vi "Read TReading.vi"(8 "error in (no error)":errorcluster, 11 "CameraSession in":refnum<class "CameraSession.lvclass">) -> (0 "error out":errorcluster, 2 "TReading":i16, 3 "CameraSession out":refnum<class "CameraSession.lvclass">)   [LabVIEW 2013, in "CameraSession.lvclass"]
uses:
  CameraSession.lvclass
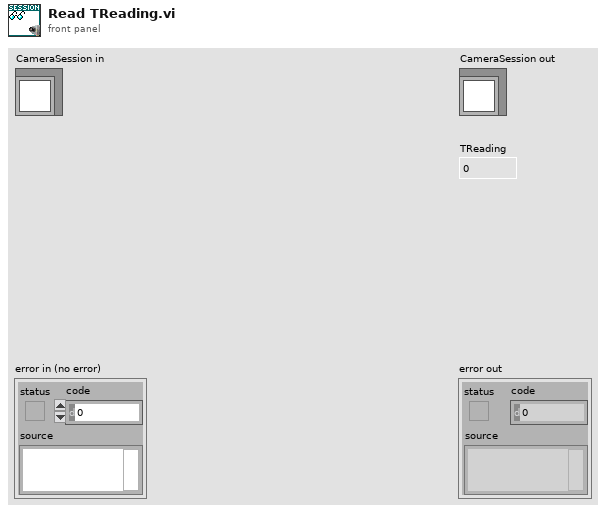
[diagram p1: front panel]
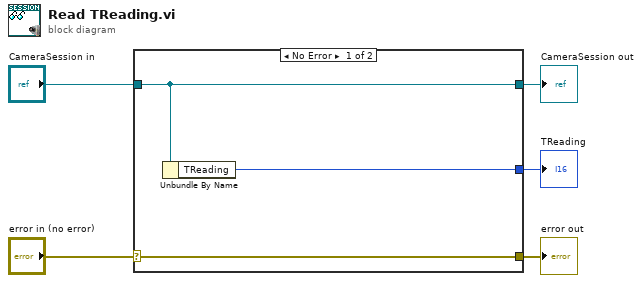
[diagram p0: block diagram]
diagram:
  n1 = case shown="No Error" "error in (no error)" {
    selector: "error in (no error)" -> [w8 w9]
    tunnel: [w8 w9] -> w4
    tunnel: [w7 w10] -> w2
    tunnel: "CameraSession in" -> [w7 w10]
    tunnel: [w6 _] -> w1
    frame No Error {
      n2 = Unbundle By Name(w7) -> ("TReading"=w6:i16)
    }
    frame Error {
    }
  }
  "error out" <- w4
  "CameraSession out" <- w2
  "TReading" <- w1
